vi "DBTimeString.vi"(4 "Time Stamp":timestamp) -> (1 "SQLite Time String":string)   [LabVIEW 2015, in "DBToolkit.lvlib"]
uses:
  DBToolkit.lvlib
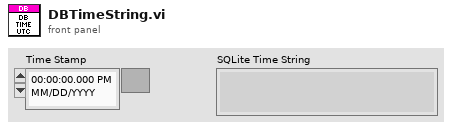
[diagram p1: front panel]
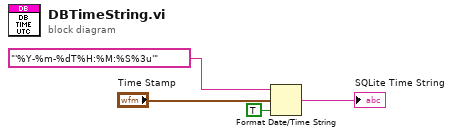
[diagram p0: block diagram]
diagram:
  n1 = Format Date/Time String(time format string (%c)="'%Y-%m-%dT%H:%M:%S%3u'", seconds (now)="Time Stamp", UTC format=TRUE) -> (date/time string=→"SQLite Time String":string)
